vi "Configure Input Settings.vi"(0 "VISA resource name":refnum<visa-resource-name>, 5 "Input (0: A)":u16(ring) items=["A", "B"], 7 "Sensor Type (0: Silicon Diode)":i8(ring) items=["Silicon Diode", "GaAIAS Diode", "100 Ohm Platinum/250", "100 Ohm Platinum/500", "1000 Ohm Platinum", "NTC RTD", "Thermo/25mV", "Thermo/50mV"], 9 "Compensation (0: Off)":i8(ring) items=["Off", "On"], 11 "error in (no error)":errorcluster, 12 "Curve Number (0)":dbl min=0.0 max=41.0 step=1.0) -> (4 "VISA resource name out":refnum<visa-resource-name>, 15 "error out":errorcluster)   [LabVIEW 2013, in "Lake Shore Cryotronics 331.lvlib"]
doc: "This VI configures the 331 input setup. The parameters configured are input type, compensation, and input curve."
uses:
  Lake Shore Cryotronics 331.lvlib
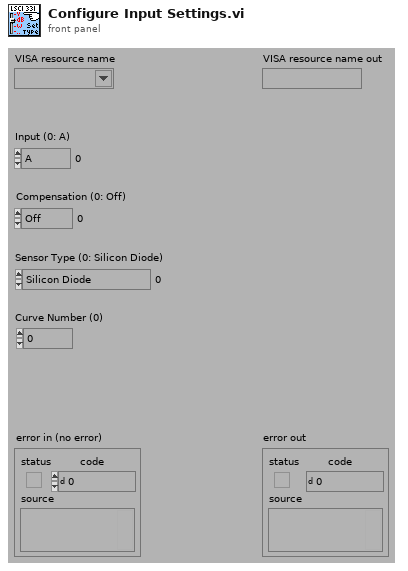
[diagram p1: front panel]
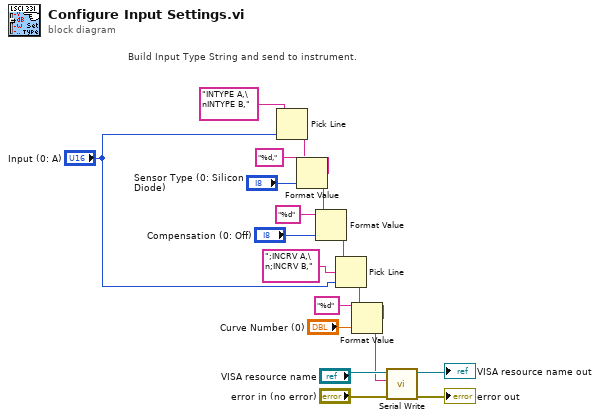
[diagram p0: block diagram]
diagram:
  # "Build Input Type String and send to instrument."
  n1 = Pick Line(multi-line string="INTYPE A,\nINTYPE B,", line index="Input (0: A)") -> (output string=w9:string)  [unwired: 1 in]
  n2 = Format Value(string ("")=w9, format string="%d,", value (0)="Sensor Type (0: Silicon Diode)") -> (output string=w7:string)
  n3 = Format Value(string ("")=w7, format string="%d", value (0)="Compensation (0: Off)") -> (output string=w5:string)
  n4 = Pick Line(string ("")=w5, multi-line string=";INCRV A,\n;INCRV B,", line index="Input (0: A)") -> (output string=w3:string)
  n5 = Format Value(string ("")=w3, format string="%d", value (0)="Curve Number (0)") -> (output string=w1:string)
  n6 = call "Serial Write.vi"("error in (no error)"="error in (no error)", "Write Buffer (\"\")"=w1, "VISA resource name"="VISA resource name") -> ("error out"=→"error out":errorcluster, "VISA resource name out"=→"VISA resource name out":refnum<visa-resource-name>)  [unwired: 6 in, 1 out]
